vi "TCP_CLIENT.vi"(7 "Timeout (ms)":i32=5000, 8 "Error In":errorcluster, 9 "Port_Number":u16=25534, 10 "IP_Address":string="192.168.0.100", 11 "TCP_In":refnum<k5>) -> (0 "error out":errorcluster, 2 "Connected?":bool, 3 "TCP_Out":refnum<k5>)   [LabVIEW 2023]
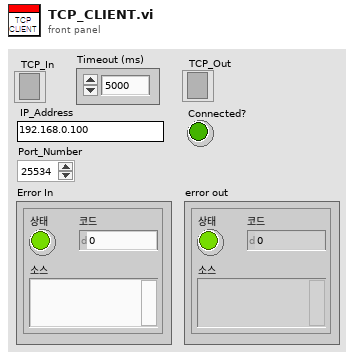
[diagram p1: front panel]
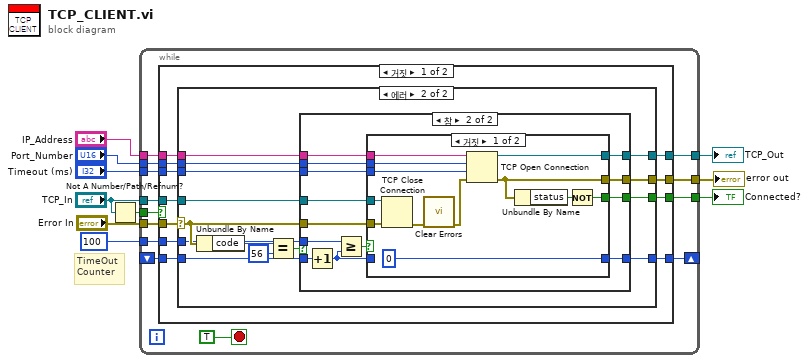
[diagram p0: block diagram]
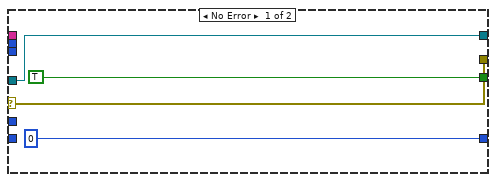
[diagram p2: hidden frame]
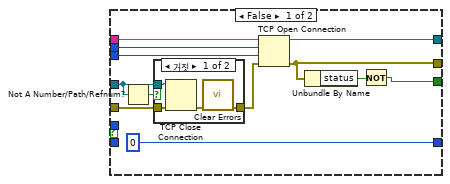
[diagram p3: hidden frame]
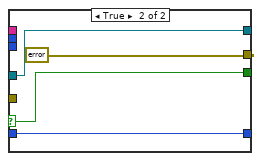
[diagram p5: hidden frame]
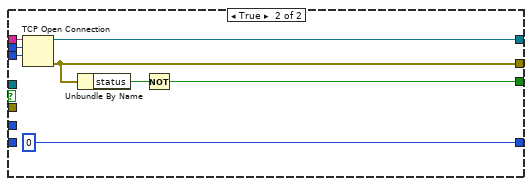
[diagram p6: hidden frame]
diagram:
  # "TimeOut\nCounter"
  n1 = Not A Number/Path/Refnum?(number/path/refnum="TCP_In") -> (NaN/Path/Refnum?=w10:bool)
  n2 = while {
    tunnel: w10 -> [w23]
    tunnel: "TCP_In" -> [w22]
    tunnel: "Error In" -> [w21]
    tunnel: "Timeout (ms)" -> [w20]
    tunnel: [w19] -> w6
    tunnel: [w18] -> w5
    tunnel: [w17] -> w4
    tunnel: "Port_Number" -> [w16]
    tunnel: "IP_Address" -> [w15]
    shift-right: [w13] -> _
    shift-left: _ -> [w12]
    tunnel: 100 ("Timeout_MaxCount") -> [w11]
    stop <- TRUE stop-if-true
    n3 = case shown="거짓" w23 {
      tunnel: w22 -> [w31 _]
      tunnel: w21 -> [w33 _]
      tunnel: w16 -> [w32 w106]
      tunnel: w15 -> [w30 w105]
      tunnel: w20 -> [w34 w104]
      tunnel: [w29 w103] -> w17
      tunnel: [w28 w101] -> w19
      tunnel: [w27 w102] -> w18
      tunnel: [w25 0] -> w13
      tunnel: w12 -> [w26 _]
      tunnel: w11 -> [w24 _]
      frame False {
        n4 = case shown="에러" w33 {
          selector: w33 -> [w37 w49]
          tunnel: w34 -> [_ w48]
          tunnel: w32 -> [_ w47]
          tunnel: w31 -> [w38 w45]
          tunnel: w30 -> [_ w46]
          tunnel: [w38 w44] -> w27
          tunnel: [w37 w43] -> w28
          tunnel: [TRUE w42] -> w29
          tunnel: w26 -> [_ w41]
          tunnel: [0 w39] -> w25
          tunnel: w24 -> [_ w40]
          frame No Error {
          }
          frame Error {
            n5 = Unbundle By Name(w49) -> ("code"=w52:i32)
            n6 = Equal?(x=w52, y=56) -> (x = y?=w50:bool)
            n7 = case shown="참" w50 {
              tunnel: w49 -> [w61 w73]
              tunnel: w48 -> [w64 w70]
              tunnel: w47 -> [w63 w71]
              tunnel: w46 -> [w62 w72]
              tunnel: w45 -> [w56 w77]
              tunnel: [w58 w78] -> w44
              tunnel: [w59 w79] -> w43
              tunnel: [w60 w74] -> w42
              tunnel: w41 -> [_ w82]
              tunnel: w40 -> [_ w81]
              tunnel: [0 w75] -> w39
              frame False {
                n8 = Not A Number/Path/Refnum?(number/path/refnum=w56) -> (NaN/Path/Refnum?=w54:bool)
                n9 = case shown="거짓" w54 {
                  tunnel: w61 -> [w67 w69]
                  tunnel: w56 -> [w68 _]
                  tunnel: [w65 w69] -> w53
                  frame False {
                    n10 = TCP Close Connection(connection ID=w68, error in (no error)=w67) -> (error out=w66:errorcluster)  [unwired: 1 in, 1 out]
                    n11 = call <vilib>:"Clear Errors.vi"("error in (no error)"=w66) -> ("error out"=w65:errorcluster)  [unwired: 5 in, 1 out]
                  }
                  frame True {
                  }
                }
                n12 = TCP Open Connection(address=w62, remote port or service name=w63, timeout ms (60000)=w64, error in (no error)=w53) -> (connection ID=w58:refnum<k5>, error out=w59:errorcluster)  [unwired: 1 in]
                n13 = Unbundle By Name(w59) -> ("status"=w55:bool)
                n14 = Not(x=w55) -> (.not. x?=w60:bool)
              }
              frame True {
                n15 = Increment(x=w82) -> (x+1=w76:i32)
                n16 = Greater Or Equal?(x=w81, y=w76) -> (x >= y?=w80:bool)
                n17 = case shown="거짓" w80 {
                  selector: w80 -> [_ w95]
                  tunnel: [w87 errorcluster {"status"=FALSE, "code"=0, "source"=""} ("error out")] -> w79
                  tunnel: [w89 w97] -> w78
                  tunnel: w77 -> [w94 w97]
                  tunnel: w76 -> [_ w96]
                  tunnel: [0 w96] -> w75
                  tunnel: [w86 w95] -> w74
                  tunnel: w73 -> [w93 _]
                  tunnel: w72 -> [w92 _]
                  tunnel: w71 -> [w91 _]
                  tunnel: w70 -> [w90 _]
                  frame False {
                    n18 = TCP Close Connection(connection ID=w94, error in (no error)=w93) -> (error out=w84:errorcluster)  [unwired: 1 in, 1 out]
                    n19 = call <vilib>:"Clear Errors.vi"("error in (no error)"=w84) -> ("error out"=w83:errorcluster)  [unwired: 5 in, 1 out]
                    n20 = TCP Open Connection(address=w92, remote port or service name=w91, timeout ms (60000)=w90, error in (no error)=w83) -> (connection ID=w89:refnum<k5>, error out=w87:errorcluster)  [unwired: 1 in]
                    n21 = Unbundle By Name(w87) -> ("status"=w85:bool)
                    n22 = Not(x=w85) -> (.not. x?=w86:bool)
                  }
                  frame True {
                  }
                }
              }
            }
          }
        }
      }
      frame True {
        n23 = TCP Open Connection(address=w105, remote port or service name=w106, timeout ms (60000)=w104) -> (connection ID=w102:refnum<k5>, error out=w101:errorcluster)  [unwired: 1 in, 1 out]
        n24 = Unbundle By Name(w101) -> ("status"=w100:bool)
        n25 = Not(x=w100) -> (.not. x?=w103:bool)
      }
    }
  }
  "error out" <- w6
  "TCP_Out" <- w5
  "Connected?" <- w4
